vi "Write Condition.vi"(8 "error in (no error)":errorcluster, 10 "Interlock Condition":bool, 11 "Interlock Bool in":refnum<class "Interlock Bool.lvclass">) -> (0 "error out":errorcluster, 3 "Interlock Bool out":refnum<class "Interlock Bool.lvclass">)   [LabVIEW 2015, in "Interlocks.lvlib" / "Interlock Bool.lvclass"]
uses:
  Interlock Bool.lvclass
  Interlock Bool.lvclass/Interlock Bool.ctl
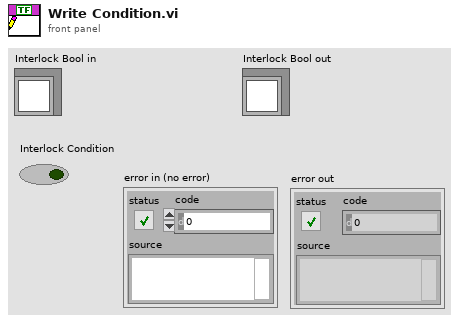
[diagram p1: front panel]
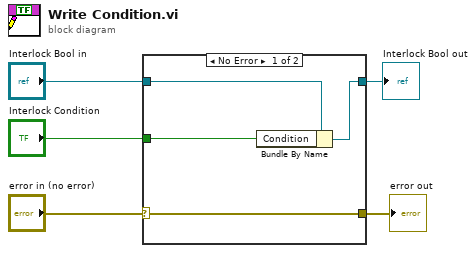
[diagram p0: block diagram]
diagram:
  n1 = case shown="No Error" "error in (no error)" {
    selector: "error in (no error)" -> [w6 w11]
    tunnel: "Interlock Bool in" -> [w9 w10]
    tunnel: [w8 w10] -> w4
    tunnel: "Interlock Condition" -> [w7 _]
    tunnel: [w6 w11] -> w1
    frame No Error {
      n2 = Bundle By Name(cluster=w9, "Condition"=w7) -> (w8:refnum<class "Interlock Bool.lvclass">)
    }
    frame Error {
    }
  }
  "Interlock Bool out" <- w4
  "error out" <- w1
